vi "Test Find Chars Separated by added chars.vi"(11 "Test Case In":refnum<class "Removed Section Finder Test.lvclass">) -> (0 "error out":errorcluster, 3 "Test Case Out":refnum<class "Removed Section Finder Test.lvclass">)   [LabVIEW 2020, in "Removed Section Finder Test.lvclass"]
uses:
  Removed Section Finder Test.lvclass
  usr/local/natinst/LabVIEW-2026-64/vi.lib/Astemes/LUnit/Test Case.lvclass
  <vilib>/Astemes/LUnit/Test Case.lvclass/Test Case.ctl
  <vilib>/Astemes/LUnit/Test Case.lvclass
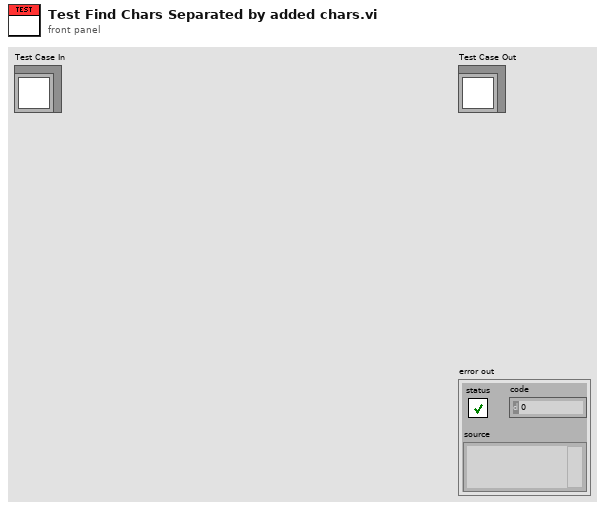
[diagram p1: front panel]
types:
  T1 = cluster{"Selection Start":u32, "Selection End":u32}[]
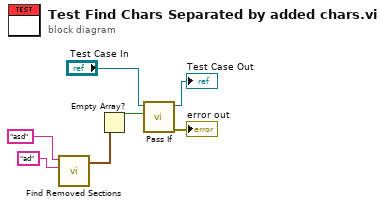
[diagram p0: block diagram]
diagram:
  n1 = call "Find Removed Sections.vi"("Reference"="ad", "Target"="asd") -> ("Sections in Reference"=w1:T1)  [unwired: 9 in]
  n2 = Empty Array?(array=w1) -> (empty?=w2:bool)
  n3 = call <vilib>:"Pass If.vi"("Pass?"=w2, "LUnit Test Case In"="Test Case In") -> ("error out"=→"error out":errorcluster, "LUnit Test Case Out"=→"Test Case Out":refnum<class "Removed Section Finder Test.lvclass">)  [unwired: 8 in]
